vi "add issue.vi"(6 "Update All (T)":bool=TRUE, 8 "error in (no error)":errorcluster, 10 "Issue Path":path, 11 "manager_daemon in":refnum<class "manager_daemon.lvclass">) -> (0 "error out":errorcluster, 3 "manager_daemon out":refnum<class "manager_daemon.lvclass">)   [LabVIEW 2024, in "manager_daemon.lvclass"]
uses:
  manager_daemon.lvclass
  type_defs/msg--cluster.ctl
  type_defs/cmd--enum.ctl
  manager_daemon.lvclass/manager_daemon.ctl
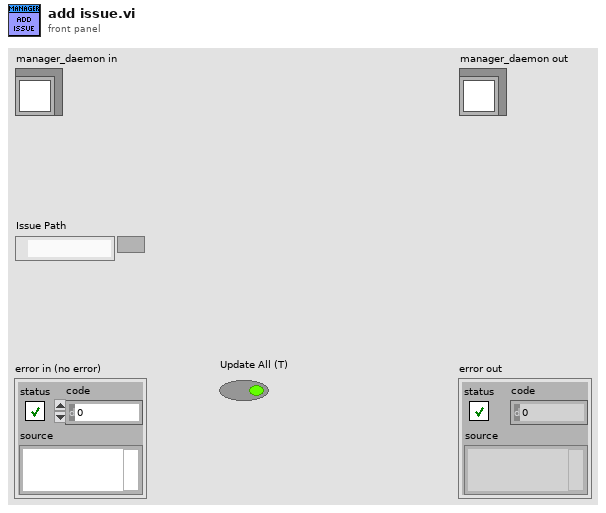
[diagram p1: front panel]
types:
  T1 = typedef "manager_daemon.lvclass/msg--cluster.ctl" = cluster{"cmd":T2, "data":variant}
  T2 = typedef "manager_daemon.lvclass/cmd--enum.ctl" = enum16{"init", "run", "load binaries", "build binaries", "save binaries", "create folder map", "display info", "apply filter", "add volume", "add issues", "add issue", "get issues", "get volume", "update volume", "delete volume", "delete issues", "exit"}
  T3 = cluster{"Issue Path":path, "Update All (T)":bool}
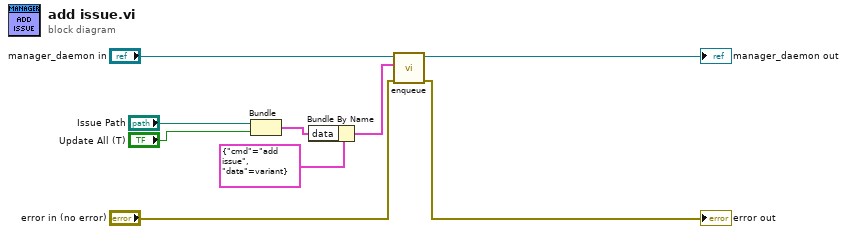
[diagram p0: block diagram]
diagram:
  n1 = Bundle("Issue Path"="Issue Path", "Update All (T)"="Update All (T)") -> (w2:T3)  [unwired: 1 in]
  n2 = Bundle By Name(cluster=T1 {"cmd"=enum."add issue", "data"=variant} ("msg"), "data"=w2) -> (w6:T1)
  n3 = call "enqueue.vi"("error in (no error)"="error in (no error)", "msg"=w6, "manager_daemon in"="manager_daemon in") -> ("error out"=→"error out":errorcluster, "manager_daemon out"=→"manager_daemon out":refnum<class "manager_daemon.lvclass">)  [unwired: 7 in]
